vi "DatabaseUISpecificInfo.vi"(0 "Model.lvclass":refnum<class "Model.lvclass">, 11 "error in (no error)":errorcluster) -> (4 "Model.lvclass  out":refnum<class "Model.lvclass">, 6 "TableName":string, 8 "TableItems":string[](array[string]), 10 "TableItemInfo":T1[](array[typedef]), 15 "error out":errorcluster)   [LabVIEW 2015, in "UserManagement.lvlib" / "Model.lvclass"]
uses:
  UserManagement/Model/Model.lvclass
  <vilib>/addons/database/Auxilliary.llb/DB Tools Column Info.ctl
  <vilib>/addons/database/Auxilliary.llb/DB Tools DataTypes.ctl
  <vilib>/addons/database/NI_Database_API.lvlib
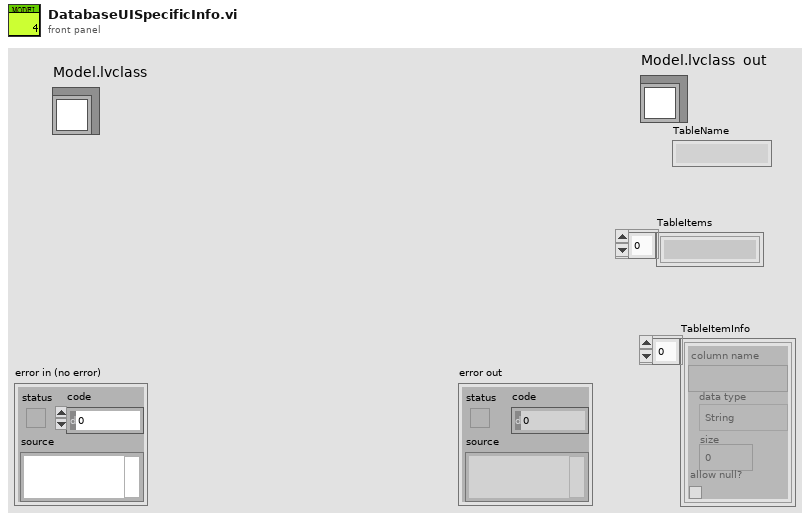
[diagram p1: front panel]
types:
  T1 = typedef "NI_Database_API.lvlib/DB Tools Column Info.ctl" = cluster{"column name":string, "data type":T2, "size":i32, "allow null?":bool}
  T2 = typedef "NI_Database_API.lvlib/DB Tools DataTypes.ctl" = enum16{"String", "Long (I32)", "Single (SGL)", "Double (DBL)", "Date/Time", "Binary"}
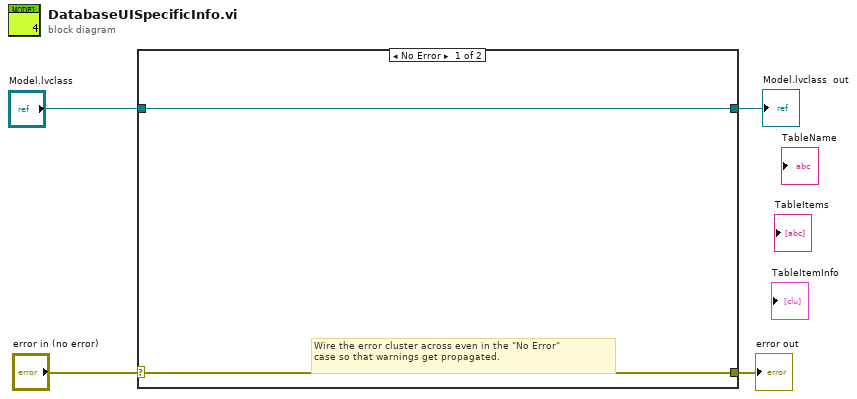
[diagram p0: block diagram]
diagram:
  n1 = case shown="No Error" "error in (no error)" {
    selector: "error in (no error)" -> [w5 w8]
    tunnel: [w5 w8] -> w3
    tunnel: [w6 w7] -> w1
    tunnel: "Model.lvclass" -> [w6 w7]
    frame No Error {
      # "Wire the error cluster across even in the \"No Error\"\ncase so that warnings get propagated."
    }
    frame Error {
    }
  }
  "error out" <- w3
  "Model.lvclass  out" <- w1
